vi "OAT Even Angle Signal Sample Rate Conversion.vi"   [LabVIEW 2017, in "SoundVib_OAUtility.lvlib"]
doc: "Converts the sample rate of the even-angle signal. Use this VI to specify a new revolution interval for sampling. Each instance of this VI maintains its own state; use the N waveforms instance of this VI to process an array of channels. Wire data to the <B>even-angle signal</B> input to determine the polymorphic instance to use or manually select the instance."
uses:
  <vilib>/addons/Sound and Vibration/Order Analysis/Utility/SoundVib_OAUtility.lvlib
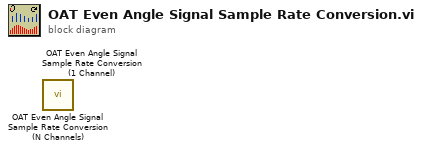
[diagram p0: block diagram]
diagram:
  n1 = call <vilib>:"OAT Even Angle Signal Sample Rate Conversion (N Channels).vi"() -> ()  [unwired: 12 in, 4 out]
  n2 = call <vilib>:"OAT Even Angle Signal Sample Rate Conversion (1 Channel).vi"() -> ()  [unwired: 12 in, 4 out]
